vi "ProcessReadings.vi"(1 "ActualValues":T1, 5 "error in (no error)":errorcluster) -> (19 "error out":errorcluster)   [LabVIEW 2019, in "IndoorData.lvclass"]
uses:
  IndoorData.lvclass
  ActualValues.ctl
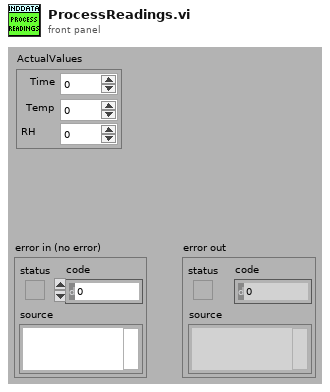
[diagram p1: front panel]
types:
  T1 = typedef "IndoorData.lvclass/ActualValues.ctl" = cluster{"Time":dbl, "Temp":dbl, "RH":dbl}
  T2 = typedef "IndoorData.lvclass/ObjectAttributes.ctl" = cluster{"DebugData":T3, "Actual":T1, "BufferedReadings":T4, "AVGReadings":T4, "LogFolder":path, "FirstLog?":bool, "MinMaxFile":path}
  T3 = typedef "IndoorData.lvclass/DebugData.ctl" = cluster{"Rev":string, "Location":string, "LoopIdx":i32, "PiCoreTemp":dbl, "Error":errorcluster}
  T4 = typedef "IndoorData.lvclass/BufferedReadings.ctl" = cluster{"Time":dbl[], "Temp":dbl[], "RH":dbl[]}
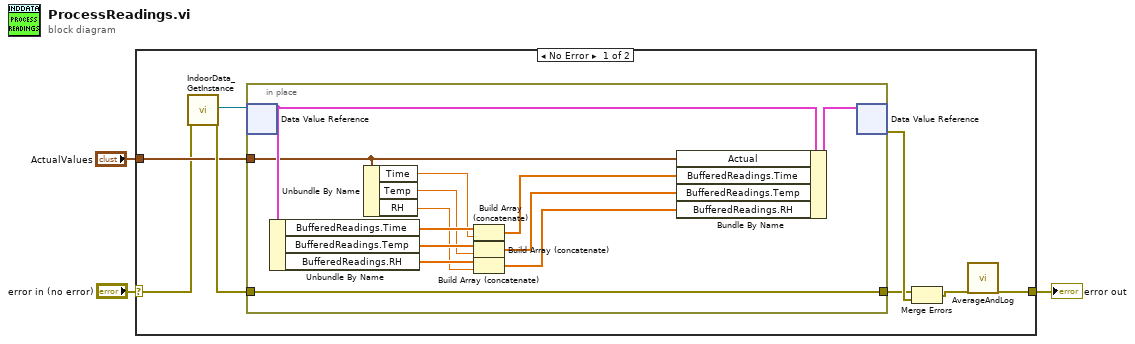
[diagram p0: block diagram]
diagram:
  n1 = case shown="No Error" "error in (no error)" {
    selector: "error in (no error)" -> [w6 w25]
    tunnel: [w4 w25] -> w2
    tunnel: "ActualValues" -> [w7 _]
    frame No Error {
      n2 = call "IndoorData_GetInstance.vi"("error in (no error)"=w6) -> ("DVRRefOut"=w10:refnum<data-value>, "error out"=w9:errorcluster)  [unwired: 14 in, 3 out]
      n3 = in-place {
        in-place-border: w9 -> [w23]
        in-place-border: [w23] -> w8
        in-place-border: w7 -> [w20]
        n4 = in-place-dvr #1(w10) -> (w22:T2)  [unwired: 1 out]
        n5 = Unbundle By Name(w22) -> ("BufferedReadings.Time"=w21:dbl[], "BufferedReadings.Temp"=w18:dbl[], "BufferedReadings.RH"=w17:dbl[])
        n6 = Unbundle By Name(w20) -> ("Time"=w19:dbl, "Temp"=w16:dbl, "RH"=w15:dbl)
        n7 = Build Array (concatenate)(w21, w19) -> (w14:dbl[])
        n8 = Build Array (concatenate)(w18, w16) -> (w13:dbl[])
        n9 = Build Array (concatenate)(w17, w15) -> (w12:dbl[])
        n10 = Bundle By Name(cluster=w22, "Actual"=w20, "BufferedReadings.Time"=w14, "BufferedReadings.Temp"=w13, "BufferedReadings.RH"=w12) -> (w24:T2)
        n11 = in-place-dvr #1(w24) -> (w11:errorcluster)  [unwired: 1 out]
      }
      n12 = Merge Errors(w8, w11) -> (w5:errorcluster)
      n13 = call "AverageAndLog.vi"("error in (no error)"=w5) -> ("error out"=w4:errorcluster)  [unwired: 18 in]
    }
    frame Error {
    }
  }
  "error out" <- w2
